vi "PH_StatusHandler.update Status Service.vi"(2 "Service ID":i32, 3 "Status":T1 items=["no info", "off/false/out", "on/true/in", "Failure", "Alarm", "Status 1", "Status 2", "Status 3"], 5 "error in (no error)":errorcluster) -> (19 "error out":errorcluster)   [LabVIEW 2014, in "PH_StatusHandler.lvlib"]
doc: "By this VI a status service can be updated. For this purpose,\n\n0: no info\n1: off/false\n2: on/true\n3: Failure\n4: Alarm\n5: Status 1\n6: Status 2\n7: Status 3\n\ncan be selected."
uses:
  PH_StatusHandler.Status.ctl
  PH_StatusHandler.lvlib
  CSlibraries-extern/DimLVEvent/LVDimInterface/LVDimInterface.lvlib
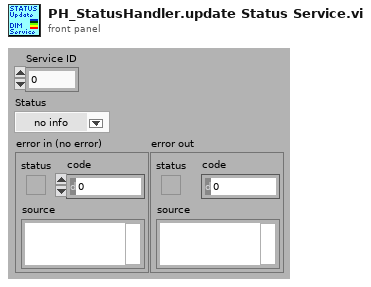
[diagram p1: front panel]
types:
  T1 = typedef "PH_StatusHandler.lvlib/PH_StatusHandler.Status.ctl" = i16
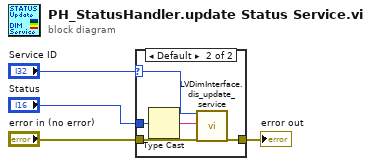
[diagram p0: block diagram]
diagram:
  n1 = case shown="Default" "Service ID" {
    selector: "Service ID" -> [_ w8]
    tunnel: [w5 w9] -> w4
    tunnel: "error in (no error)" -> [w5 w10]
    tunnel: "Status" -> [_ w6]
    frame -1 {
    }
    frame Default {
      n2 = Type Cast(x=w6) -> (*(type *) &x=w7:string)  [unwired: 1 in]
      n3 = call "LVDimInterface.dis_update_service.vi"("my_serviceID"=w8, "data"=w7, "error in (no error)"=w10) -> ("error out"=w9:errorcluster)  [unwired: 14 in, 2 out]
    }
  }
  "error out" <- w4
